vi "DI mnoz wartosci cyfrowe.vi"(6 "Mnozniki in":dbl[](array[numeric]), 7 "#cores (1)":i32=1, 8 "error in (no error)":errorcluster, 10 "Kanaly in":T1) -> (0 "error out":errorcluster, 2 "Kanaly out":T1, 5 "Niezgodnosc rozmiarow?":bool)   [LabVIEW 2013]
doc: "Mnoży wartości na aktywnych kanałach cyfrowych\nprzez mnożniki podane w konfiguracji kanalow"
uses:
  Kontrolki/Przetwarzanie/Kanaly.ctl
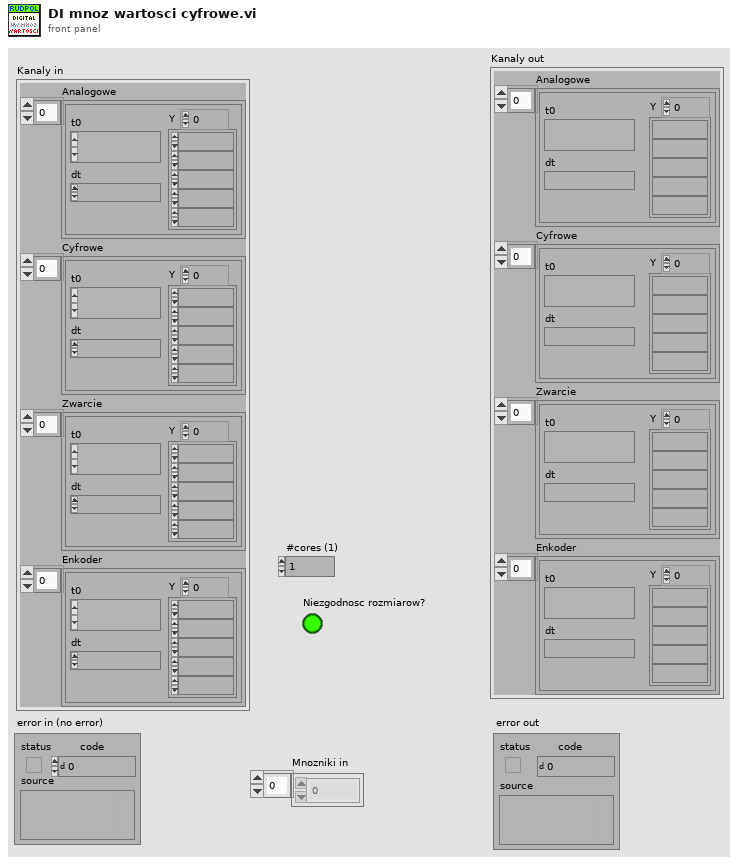
[diagram p1: front panel]
types:
  T1 = typedef "Kanaly.ctl" = cluster{"Analogowe":waveform(dbl)[], "Cyfrowe":waveform(dbl)[], "Zwarcie":waveform(dbl)[], "Enkoder":waveform(dbl)[]}
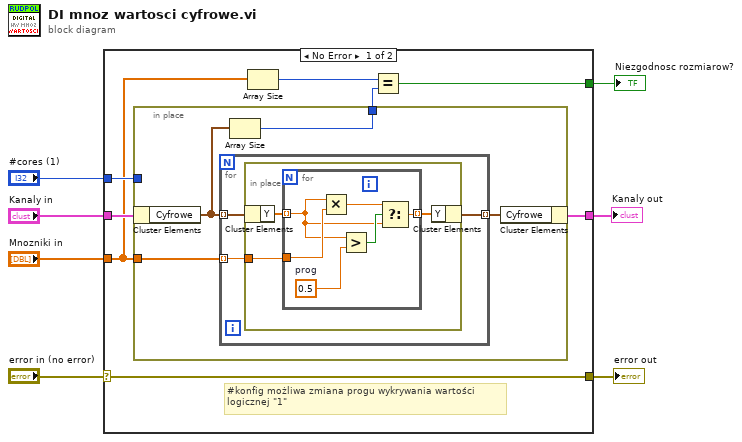
[diagram p0: block diagram]
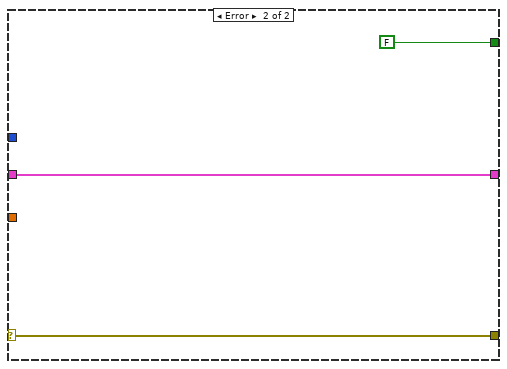
[diagram p2: hidden frame]
diagram:
  n1 = case shown="No Error" "error in (no error)" {
    selector: "error in (no error)" -> [w8 w34]
    tunnel: [w8 w34] -> w6
    tunnel: "Kanaly in" -> [w13 w32]
    tunnel: "#cores (1)" -> [w12 _]
    tunnel: "Mnozniki in" -> [w11 _]
    tunnel: [w10 FALSE] -> w2
    tunnel: [w9 w32] -> w1
    frame No Error {
      # "#konfig możliwa zmiana progu wykrywania wartości\nlogicznej \"1\""
      n2 = in-place {
        in-place-border: w11 -> [w19]
        in-place-border: [w17] -> w15
        in-place-border: w12 -> [_]
        n3 = in-place-cluster #1(w13) -> ("Cyfrowe"=w18:waveform(dbl)[])
        n4 = for {
          tunnel: w18 -> [w22] mode=indexing
          tunnel: w19 -> [w21] mode=indexing
          tunnel: [w20] -> w16 mode=indexing
          n5 = in-place {
            in-place-border: w21 -> [w25]
            n6 = in-place-cluster #2(w22) -> ("Y"=w23:dbl[])
            n7 = for {
              tunnel: w25 -> [w29]
              tunnel: [w31] -> w24 mode=indexing
              tunnel: w23 -> [w27] mode=indexing
              w26 = 0.5  # prog
              n8 = Multiply(x=w27, y=w29) -> (x*y=w30:dbl)
              n9 = Greater?(x=w27, y=w26) -> (0:w28:bool)
              n10 = Select(t=w30, s=w28, f=w27) -> (s? t:f=w31:dbl)
            }
            n11 = in-place-cluster #2("Y"=w24) -> (w20:waveform(dbl))
          }
        }
        n12 = Array Size(array=w18) -> (size(s)=w17:i32)
        n13 = in-place-cluster #1("Cyfrowe"=w16) -> (w9:T1)
      }
      n14 = Array Size(array=w11) -> (size(s)=w14:i32)
      n15 = Equal?(x=w14, y=w15) -> (x = y?=w10:bool)
    }
    frame Error {
    }
  }
  "error out" <- w6
  "Kanaly out" <- w1
  "Niezgodnosc rozmiarow?" <- w2
